vi "Arrays Data and importing.vi"() -> ()   [LabVIEW 2019, in "OPI.lvclass"]
uses:
  OPI.lvclass
  Typedefs/Cmd Line Mode.ctl
  Set Arguments/Set Argument - Integer.vi
  Get Return/Get Return - Integer Array.vi
panel:
  out "Return Data":i64[](graph)=[4, 7, 9, 0, 3, 2, 3, 7, 0, 6, 4, 8, 7, 1, 8, 7, 5, 6, 5, 8, 7, 7, 8, 8, 0, 5, 5, 4, 8, 7, 0, 8, 0, 10, 3, 6, 3, 0, 0, 9, 1, 6, 4, 1, 5, 3, 10, 0, 3, 9, 3, 1, 9, 0, 4, 0, 6, 9, 10, 4, 0, 1, 0, 7, 5, 5, 10, 8, 8, 10, 3, 6, 1, 3, 0, 0, 4, 1, 3, 10, 8, 0, 4, 8, 10, 6, 0, 1, 5, 7, 8, 8, 6, 6, 9, 5, 8, 5, 7, 3]
  in  "Amplitude":i64=10
  in  "# Samples":i64=100
  in  "Stop":bool
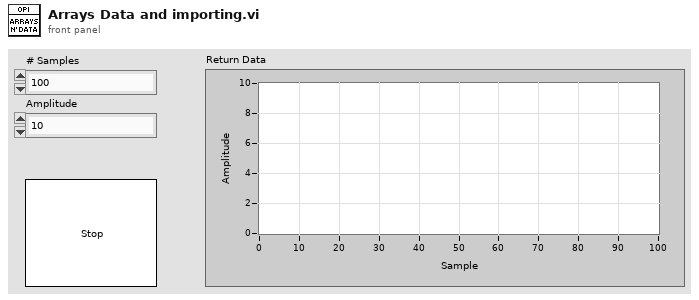
[diagram p1: front panel]
types:
  T1 = typedef "OPI.lvclass/Cmd Line Mode.ctl" = enum16{"Debug", "Hidden"}
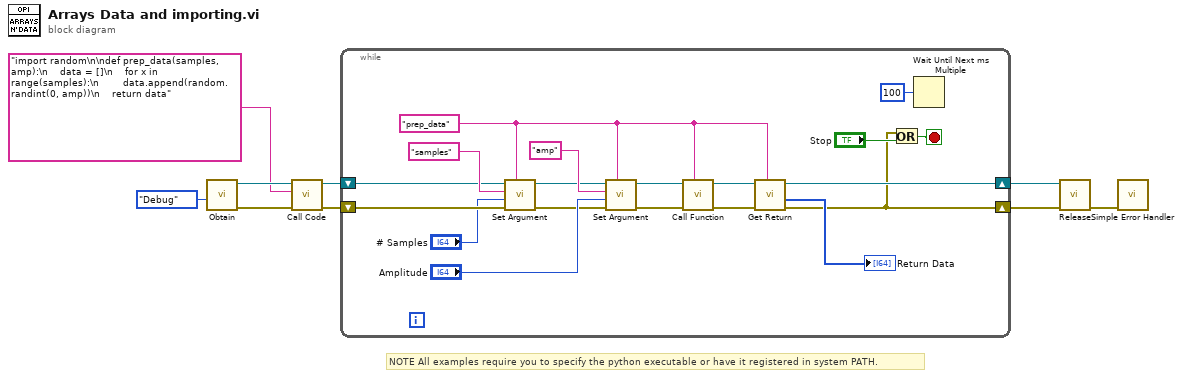
[diagram p0: block diagram]
diagram:
  # "NOTE All examples require you to specify the python executable or have it registered in system PATH."
  n1 = call "Obtain.vi"("Cmd Line Mode (Hidden)"=Cmd_Line_Mode."Debug") -> ("Error Out"=w8:errorcluster, "OPI Ref"=w9:refnum<data-value>)  [unwired: 9 in]
  n2 = call "Call Code.vi"("Error In"=w8, "Pythonic Code"="import random\n\ndef prep_data(samples, amp):\n    data = []\n    for x in range(samples):\n        data.append(random.randint(0, amp))\n    return data", "OPI Ref"=w9) -> ("Error Out"=w5:errorcluster, "OPI Ref"=w6:refnum<data-value>)  [unwired: 7 in]
  n3 = while {
    shift-right: [w11] -> w4
    shift-left: w6 -> [w13]
    shift-right: [w10] -> w2
    shift-left: w5 -> [w16]
    stop <- w28 stop-if-true
    w19 = "prep_data" ("Function Name")
    n4 = call-poly "Set Argument.vi"("Function Name"=w19, "Error In"=w16, "Integer"="# Samples", "Argument"="samples" ("Function Name"), "OPI Ref"=w13) -> ("Error Out"=w17:errorcluster, "OPI Ref"=w18:refnum<data-value>)  [unwired: 5 in]
    n5 = call-poly "Set Argument.vi"("Function Name"=w19, "Error In"=w17, "Integer"="Amplitude", "Argument"="amp" ("Function Name"), "OPI Ref"=w18) -> ("Error Out"=w22:errorcluster, "OPI Ref"=w23:refnum<data-value>)  [unwired: 5 in]
    n6 = call "Call Function.vi"("Function Name"=w19, "Error In"=w22, "OPI Ref"=w23) -> ("Error Out"=w24:errorcluster, "OPI Ref"=w25:refnum<data-value>)  [unwired: 7 in]
    n7 = call-poly "Get Return.vi"("Function Name"=w19, "Error In"=w24, "OPI Ref"=w25) -> ("Error Out"=w10:errorcluster, "Integer Array"=→"Return Data":i64[], "OPI Ref"=w11:refnum<data-value>)  [unwired: 6 in]
    n8 = Or(x=w10, y="Stop") -> (x .or. y?=w28:bool)
    n9 = Wait Until Next ms Multiple(millisecond multiple=u32 100) -> ()  [unwired: 1 out]
  }
  n10 = call "Release.vi"("Error In"=w2, "OPI Ref"=w4) -> ("Error Out"=w1:errorcluster)  [unwired: 9 in]
  n11 = call <vilib>:"Simple Error Handler.vi"("error in (no error)"=w1) -> ()  [unwired: 4 in, 5 out]
